vi "keccak.fpga.step.4.5.6.7.vi"(9 "E.Parameters":T1[](array[typedef]), 10 "D.in":u64[](array[numeric])=[0, 0, 0, 0, 0] format="%.0x", 11 "state[24]":u64[](array[numeric])=[0, 0, 0, 0, 0, 0, 0, 0, 0, 0, 0, 0, 0, 0, 0, 0, 0, 0, 0, 0, 0, 0, 0, 0] format="%.0x") -> (3 "Exy.out":u64[](array[numeric]) format="%.0x")   [LabVIEW 2021]
uses:
  host.impl/Step.4.5.6.7.Inputs.ctl
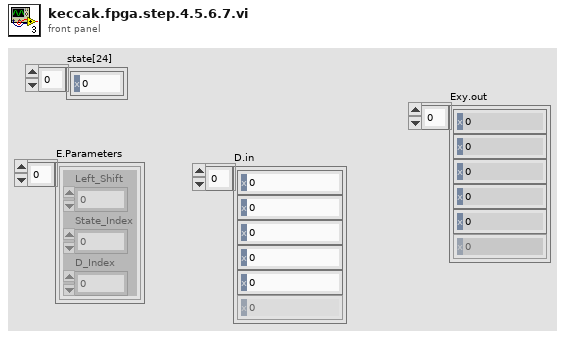
[diagram p1: front panel]
types:
  T1 = typedef "Step.4.5.6.7.Inputs.ctl" = cluster{"Left_Shift":i32, "State_Index":i32, "D_Index":i32}
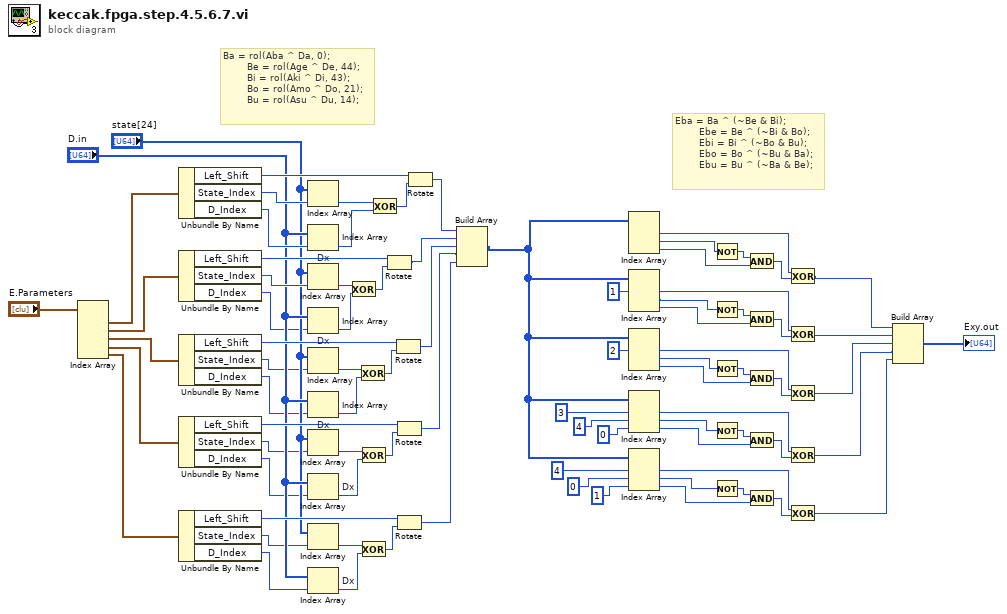
[diagram p0: block diagram]
diagram:
  # "Ba = rol(Aba ^ Da, 0);\n        Be = rol(Age ^ De, 44);\n        Bi = rol(Aki ^ Di, 43);\n        Bo = rol(Amo ^ Do, 21);\n        Bu = rol(Asu ^ Du, 14);"
  # "Eba = Ba ^ (~Be & Bi);\n        Ebe = Be ^ (~Bi & Bo);\n        Ebi = Bi ^ (~Bo & Bu);\n        Ebo = Bo ^ (~Bu & Ba);\n        Ebu = Bu ^ (~Ba & Be);"
  n1 = Index Array(array="E.Parameters") -> (element #1=w82:T1, element #2=w74:T1, element #3=w73:T1, element #4=w72:T1, element #5=w71:T1)  [unwired: 5 in]
  n2 = Unbundle By Name(w82) -> ("Left_Shift"=w79:i32, "State_Index"=w80:i32, "D_Index"=w78:i32)
  n3 = Unbundle By Name(w74) -> ("Left_Shift"=w54:i32, "State_Index"=w50:i32, "D_Index"=w44:i32)
  n4 = Unbundle By Name(w73) -> ("Left_Shift"=w53:i32, "State_Index"=w45:i32, "D_Index"=w43:i32)
  n5 = Unbundle By Name(w72) -> ("Left_Shift"=w52:i32, "State_Index"=w46:i32, "D_Index"=w42:i32)
  n6 = Unbundle By Name(w71) -> ("Left_Shift"=w51:i32, "State_Index"=w47:i32, "D_Index"=w41:i32)
  n7 = Index Array(array="state[24]", index=w80) -> (element=w75:u64)
  n8 = Index Array "Dx"(array="D.in", index=w78) -> (element=w77:u64)
  n9 = Index Array(array="state[24]", index=w50) -> (element=w68:u64)
  n10 = Index Array "Dx"(array="D.in", index=w44) -> (element=w70:u64)
  n11 = Index Array(array="state[24]", index=w45) -> (element=w65:u64)
  n12 = Index Array "Dx"(array="D.in", index=w43) -> (element=w67:u64)
  n13 = Index Array(array="state[24]", index=w46) -> (element=w62:u64)
  n14 = Index Array "Dx"(array="D.in", index=w42) -> (element=w64:u64)
  n15 = Index Array(array="state[24]", index=w47) -> (element=w59:u64)
  n16 = Index Array "Dx"(array="D.in", index=w41) -> (element=w61:u64)
  n17 = Exclusive Or(1:w70, 2:w68) -> (0:w69:u64)
  n18 = Exclusive Or(1:w67, 2:w65) -> (0:w66:u64)
  n19 = Exclusive Or(1:w64, 2:w62) -> (0:w63:u64)
  n20 = Exclusive Or(1:w61, 2:w59) -> (0:w60:u64)
  n21 = Exclusive Or(1:w77, 2:w75) -> (0:w76:u64)
  n22 = Rotate(1:w69, 2:w54) -> (0:w58:u64)
  n23 = Rotate(1:w66, 2:w53) -> (0:w57:u64)
  n24 = Rotate(1:w63, 2:w52) -> (0:w56:u64)
  n25 = Rotate(1:w60, 2:w51) -> (0:w55:u64)
  n26 = Rotate(1:w76, 2:w79) -> (0:w83:u64)
  n27 = Build Array(w83, w58, w57, w56, w55) -> (w25:u64[])
  n28 = Index Array(array=w25) -> (element #1=w38:u64, element #2=w10:u64, element #3=w9:u64)  [unwired: 3 in]
  n29 = Index Array(array=w25, index #1=1 ("index")) -> (element #1=w35:u64, element #2=w7:u64, element #3=w8:u64)  [unwired: 2 in]
  n30 = Index Array(array=w25, index #1=2 ("index")) -> (element #1=w32:u64, element #2=w5:u64, element #3=w6:u64)  [unwired: 2 in]
  n31 = Index Array(array=w25, index #1=3 ("index"), index #2=4 ("index"), index #3=0 ("index")) -> (element #1=w29:u64, element #2=w4:u64, element #3=w3:u64)
  n32 = Index Array(array=w25, index #1=4 ("index"), index #2=0 ("index"), index #3=1 ("index")) -> (element #1=w26:u64, element #2=w1:u64, element #3=w2:u64)
  n33 = Not(x=w10) -> (.not. x?=w40:u64)
  n34 = Not(x=w7) -> (.not. x?=w37:u64)
  n35 = Not(x=w5) -> (.not. x?=w34:u64)
  n36 = Not(x=w4) -> (.not. x?=w31:u64)
  n37 = Not(x=w1) -> (.not. x?=w28:u64)
  n38 = And(x=w40, y=w9) -> (x .and. y?=w39:u64)
  n39 = And(x=w37, y=w8) -> (x .and. y?=w36:u64)
  n40 = And(x=w34, y=w6) -> (x .and. y?=w33:u64)
  n41 = And(x=w31, y=w3) -> (x .and. y?=w30:u64)
  n42 = And(x=w28, y=w2) -> (x .and. y?=w27:u64)
  n43 = Exclusive Or(1:w39, 2:w38) -> (0:w16:u64)
  n44 = Exclusive Or(1:w36, 2:w35) -> (0:w15:u64)
  n45 = Exclusive Or(1:w33, 2:w32) -> (0:w14:u64)
  n46 = Exclusive Or(1:w30, 2:w29) -> (0:w13:u64)
  n47 = Exclusive Or(1:w27, 2:w26) -> (0:w12:u64)
  n48 = Build Array(w16, w15, w14, w13, w12) -> (→"Exy.out":u64[])
